vi "LaserCal-Save Data (Dynamic).vi"(0 "System ID":T1, 7 "I-O Data":T2, 11 "error in (no error)":errorcluster) -> (15 "error out":errorcluster)   [LabVIEW 2015]
uses:
  Typedefs/LaserCal-Data (Dynamic).ctl
  Typedefs/LaserCal-System ID.ctl
panel:
  in  "Laser Dynamic Calibration File":T3
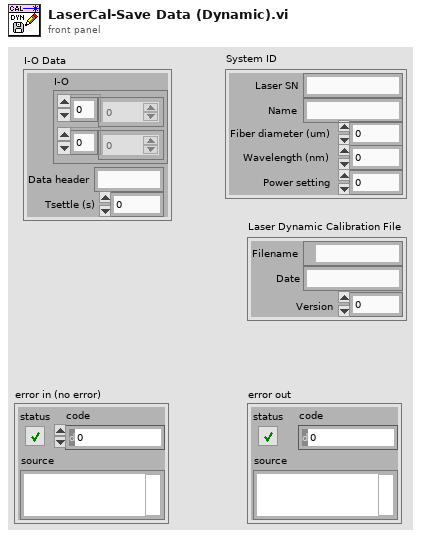
[diagram p1: front panel]
types:
  T1 = typedef "LaserCal-System ID.ctl" = cluster{"Name":string, "Laser SN":string, "Wavelength (nm)":dbl, "Fiber diameter (um)":dbl, "Power setting":dbl}
  T2 = typedef "LaserCal-Data (Dynamic).ctl" = cluster{"I-O":cluster{dbl[], dbl[]}, "Data header":string, "Tsettle (s)":dbl}
  T3 = cluster{"Filename":path, "Date":string, "Version":i32}
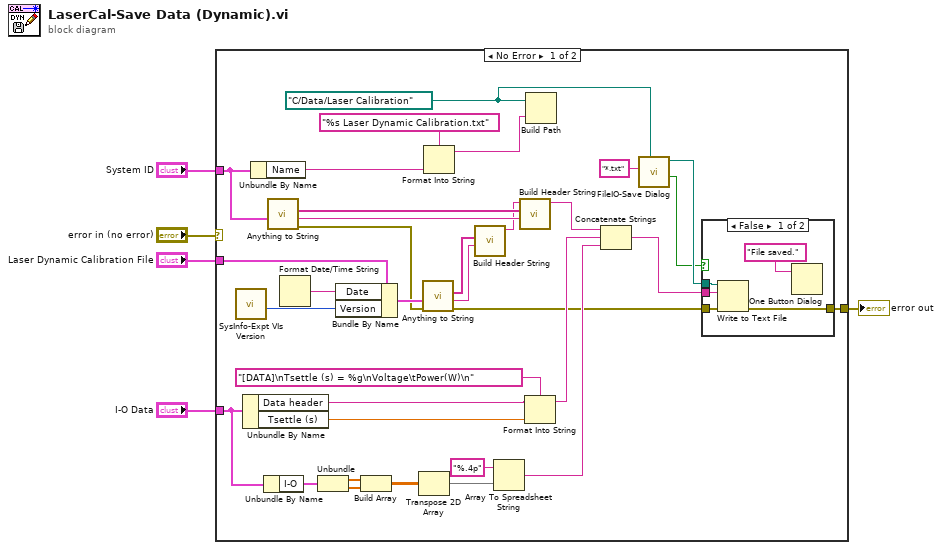
[diagram p0: block diagram]
diagram:
  n1 = case shown="No Error" "error in (no error)" {
    selector: "error in (no error)" -> [_ w46]
    tunnel: [w14 w46] -> w5
    tunnel: "Laser Dynamic Calibration File" -> [w37 _]
    tunnel: "I-O Data" -> [w12 _]
    tunnel: "System ID" -> [w18 _]
    frame No Error {
      w10 = path "C:/Data/Laser Calibration"
      n2 = call "SysInfo-Expt VIs Version.vi"() -> ("Expt VIs Version out"=w38:i32)  [unwired: 11 in]
      n3 = Unbundle By Name(w12) -> ("Data header"=w26:string, "Tsettle (s)"=w27:dbl)
      n4 = Unbundle By Name(w18) -> ("Name"=w17:string)
      n5 = Unbundle By Name(w12) -> ("I-O"=w33:cluster{dbl[], dbl[]})
      n6 = call "Anything to String.vi"("Anything"=w18) -> ("Error Out"=w22:errorcluster, "Section"=w23:string, "Strings[]"=w21:string[])  [unwired: 8 in]
      n7 = Format Date/Time String() -> (date/time string=w39:string)  [unwired: 3 in]
      n8 = Unbundle(w33) -> (w32:dbl[], w31:dbl[])
      n9 = Bundle By Name(cluster=w37, "Date"=w39, "Version"=w38) -> (w36:T3)
      n10 = Build Array(w32, w31) -> (w30:dbl[][])
      n11 = Transpose 2D Array(2D array=w30) -> (transposed array=w11:dbl[][])
      n12 = call "Anything to String.vi"("Error In"=w22, "Anything"=w36) -> ("Error Out"=w9:errorcluster, "Section"=w34:string, "Strings[]"=w35:string[])  [unwired: 7 in]
      n13 = Format Into String(format string="%s Laser Dynamic Calibration.txt", w17) -> (resulting string=w15:string)  [unwired: 2 in, 1 out]
      n14 = call "Build Header String.vi"("Section"=w34, "Strings[]"=w35) -> ("Header out"=w20:string)  [unwired: 9 in]
      n15 = Array To Spreadsheet String(array=w11, 3:"%.4p" ("format string")) -> (spreadsheet string=w24:string)  [unwired: 1 in]
      n16 = call "Build Header String.vi"("Section"=w23, "Strings[]"=w21, "Header in"=w20) -> ("Header out"=w19:string)  [unwired: 8 in]
      n17 = Format Into String(format string="[DATA]\nTsettle (s) = %g\nVoltage\tPower(W)\n", initial string=w26, w27) -> (resulting string=w25:string)  [unwired: 1 in, 1 out]
      n18 = Build Path(base path=w10, name or relative path=w15) -> ()  [unwired: 1 out]
      n19 = Concatenate Strings(w19, w25, w24) -> (w13:string)
      n20 = call "FileIO-Save Dialog.vi"("Default Folder"=w10, "pattern (all files)"="*.txt") -> ("cancelled"=w7:bool, "selected path"=w8:path)  [unwired: 7 in, 1 out]
      n21 = case shown="False" w7 {
        tunnel: [w44 w45] -> w14
        tunnel: w13 -> [w43 _]
        tunnel: w9 -> [w42 w45]
        tunnel: w8 -> [w41 _]
        frame False {
          n22 = Write to Text File(file (use dialog)=w41, text=w43, error in=w42) -> (error out=w44:errorcluster)  [unwired: 1 in, 2 out]
          n23 = One Button Dialog(message="File saved.") -> ()  [unwired: 1 in, 1 out]
        }
        frame True {
        }
      }
    }
    frame Error {
    }
  }
  "error out" <- w5
